vi "5 - select sub patterns.vi"(9 "Number of transitions":i32, 11 "All Sub patterns":string[](array[string])) -> (2 "sub patterns out":string[](array[string]))   [LabVIEW 2013]
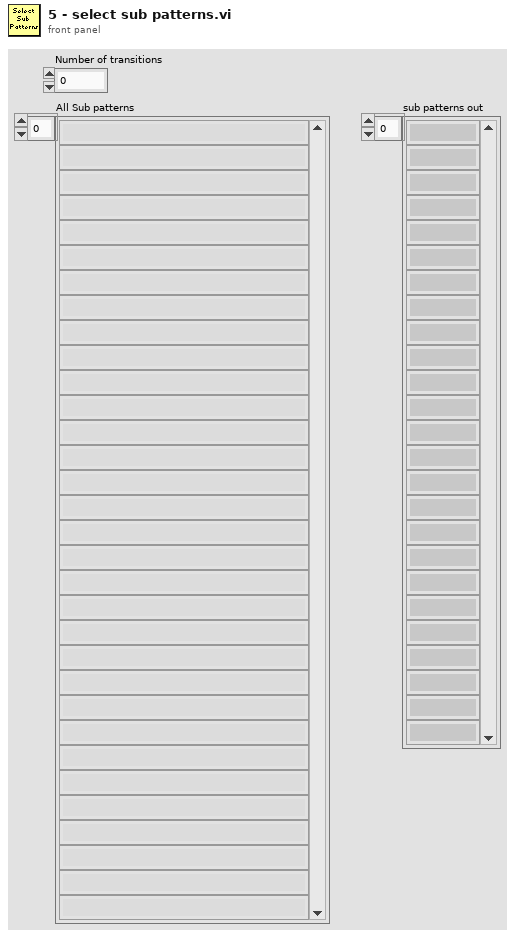
[diagram p1: front panel]
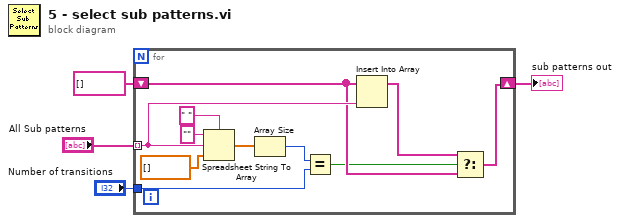
[diagram p0: block diagram]
diagram:
  n1 = for {
    tunnel: "All Sub patterns" -> [w9] mode=indexing
    tunnel: "Number of transitions" -> [w10]
    shift-right: [w6] -> w2
    shift-left: string[] [] -> [w7]
    n2 = Spreadsheet String To Array(delimiter (Tab)=" ", format string="", spreadsheet string=w9, array type (2D Dbl)=dbl[] []) -> (array=w12:dbl[])
    n3 = Array Size(array=w12) -> (size(s)=w11:i32)
    n4 = Equal?(x=w11, y=w10) -> (x = y?=w5:bool)
    n5 = Insert Into Array(array=w7, new element=w9) -> (w8:string[])  [unwired: 1 in]
    n6 = Select(t=w8, s=w5, f=w7) -> (s? t:f=w6:string[])
  }
  "sub patterns out" <- w2
